vi "AlliGator Parameter Map Actions.vi"(0 "AlliGator Q Elements in":T6[](array[typedef]), 1 "VI in":refnum<vi>, 2 "Script in":bool, 5 "data value reference":refnum<data-value>, 7 "AlliGator Q Event in":T7=enum."GUI:Idle", 9 "Data":variant, 11 "error in (no error)":errorcluster, 12 "AlliGator Ctrl Refnums":T8) -> (3 "Script out":bool, 4 "AlliGator Q Elements out":T6[](array[typedef]), 6 "Data Value Reference out":refnum<data-value>, 10 "[Notebook Message]":T1[](array[typedef]) {"Message Style"."Font Size" min=6.0 step=1.0}, 15 "error out":errorcluster)   [LabVIEW 2021, in "AlliGator Action Engine.lvlib"]
doc: "Processes AlliGator decay fit parameter map-related actions."
uses:
  AlliGator Action Engine.lvlib
  Internal Variables/AlliGator Internal Variables v2.ctl
  <vilib>/vision/Image Controls.llb/IMAQ Image.ctl
  Internal Variables/AlliGator Gate Image Set.ctl
  Files/AlliGator FLI Dataset Type.ctl
  Files/AlliGator Data Series Type.ctl
  Dual-Channel Datasets/AlliGator Dataset Channel.ctl
  Settings/AlliGator Gate Arithmetic.ctl
  Source Image/AlliGator Displayed Image.ctl
  Image/Named ROI Description.ctl
  Phasor Graph/AlliGator Decay Metadata v3.ctl
  Decay Analysis/Decay Preprocessing/AlliGator Decay Background Subtraction Info.ctl
  Decay Analysis/Decay Preprocessing/AlliGator Baseline Subtraction Method.ctl
  Graphs/XY Graph/XY Graph Plot Shift Parameters.ctl
  Graphs/XY Graph/XY Graph Plot Shift Method.ctl
  Decay Analysis/Decay Preprocessing/AlliGator Decay Extrapolation Parameters.ctl
  Phasor/Calibration Phasor (m, phi).ctl
  Phasor/Phasor Reference Series.ctl
  Phasor/Phasor Calibration Map v2.ctl
  Phasor/Phasor (g, s).ctl
  Phasor Graph/AlliGator Raw Phasor Plot Data v5.ctl
  Phasor/Phasor Standard Deviation Options.ctl
  Phasor Plot/AlliGator Phasor Multi-Harmonic Data.ctl
  Phasor/Phasor Harmonic Data.ctl
  Decay Fit Parameter Map/AlliGator Decay Fit Options & Parameters v4.ctl
  Fits/IRF(X)PSED/Decay Fit Options v4.ctl
  Fits/Decay Convolution/Decay Model.ctl
  Fits/Residual Type.ctl
  Fits/IRF(X)PSED/Fit Weights Type v2.ctl
  Fits/Non-linear Fitting Method v2.ctl
  Fits/Fit Calculation Method.ctl
  Fits/Non-linear Fitting Algorithm.ctl
  Decay Analysis/Decay Fit/AlliGator Decay Fit Parameter Constraints 2.ctl
  Fits/IRF(X)PSED/Decay Fit Parameters In List.ctl
  Fits/IRF(X)PSED/MLE Baseline Offset Type.ctl
  Decay Analysis/Decay Preprocessing/AlliGator Decay Preprocessing Parameters.ctl
  Fits/IRF(X)PSED/Decay Fit Parameters & Derived Quantities List v2.ctl
  Fits/IRF(X)PSED/Decay Fit Result Constraint.ctl
  Decay Fit Parameter Map/AlliGator Parameter Maps Data.ctl
  AlliGator Q Event.ctl
  GUI/AlliGator Ctrl Refnums.ctl
  GUI/AlliGator Other Ctrl Refnums.ctl
  GUI/AlliGator State Indicator.ctl
  GUI/AlliGator Main Window Tabs.ctl
  GUI/AlliGator Phasor Plot Ctrl Refnums.ctl
  GUI/AlliGator Phasor Graph Ctrl Refnums.ctl
  Phasor/Phasor Calibration Type.ctl
  GUI/AlliGator Dataset Ctrl Refnums.ctl
  GUI/AlliGator Registered Events Ctrl Refnums.ctl
  GUI/AlliGator Image Histogram Control Refnums.ctl
  Histograms/Linear Histogram Options.ctl
  Histograms/Histogram Bin Option.ctl
  Histograms/Histogram Bin Position.ctl
  Decay Fit Parameter Map/AlliGator Decay Fit Map Control Refnums.ctl
  Parameter Map/AlliGator Parameter Map Control Refnums.ctl
  AlliGator Q Element.ctl
  Notebook/Notebook Message Object.ctl
  Rich Text Box/Text Formatting.ctl
  Rich Text Box/Text Colors.ctl
  Rich Text Box/Text Style.ctl
  Rich Text Box/Text Alignment.ctl
  Parameter Map/AlliGator New Parameter Map Set Event Data.ctl
  Alligator Elements Order in Action Stack.ctl
  Globals, Variables, Constants/AlliGator Variables List.ctl
  GUI/AlliGator Image Display Type.ctl
  Palette/Image Palette Information.ctl
  Image/Image Display Palette Type.ctl
  Utilities/Read-Write.ctl
  GUI/AlliGator Image Mouse Up Event Data.ctl
  Image/Image ROI Descriptor.ctl
  Image/Image Contour Definition.ctl
  Image/Image Contour ID.ctl
  Image/Image ROI Type.ctl
  Image/Image Control Refnum.ctl
  Rich Text Box/Text Format List.ctl
  c5217346-0728-4db9-a30e-52dae72b7cfc.vi
  AlliGator Add Single Action to Stack.vi
  Variant/Variant to Data/Variant to [String].vi
  Variant/Variant to Data/Variant to String.vi
  Variant/Variant to Data/Variant to Boolean.vi
  Variant/Variant to Data/Variant to I32.vi
  Variant/Variant to Data/Variant to U16.vi
  GUI/GUI.lvlib
  Variant/Variant to Data/Variant to Data.lvlib
  Globals, Variables, Constants/AlliGator Globals, Variables & Constants.lvlib
  Palette/Palette.lvlib
  GUI/AlliGator GUI.lvlib
  Image/Image.lvlib
  Files/AlliGator Files.lvlib
  Internal Variables/AlliGator Internal Variables.lvlib
  Files/Load-Save File Info.ctl
  Files/Files.lvlib
  Decay Fit Parameter Map/AlliGator Decay Fit Parameter Map.lvlib
  Sound/Sound.lvlib
  Parameter Map/AlliGator Parameter Map.lvlib
  Local Decay Window/AlliGator Local Decay Window.lvlib
  Notebook/Notebook.lvlib
  Utilities/Utilities.lvlib
  Phasor/Phasor.lvlib
  Decay Analysis/Decay Preprocessing/AlliGator Decay Preprocessing.lvlib
  Graphs/XY Graph/XY Graph Add-Ons.lvlib
  Phasor Graph/AlliGator Phasor Graph.lvlib
  Phasor Plot/AlliGator Phasor Plot.lvlib
  Source Image/AlliGator Source Image.lvlib
  Fits/Fits.lvlib
  Decay Analysis/Decay Fit/AlliGator Decay Fit.lvlib
  Settings/AlliGator Settings.lvlib
  Rich Text Box/Rich Text Box.lvlib
  Dual-Channel Datasets/AlliGator Dual-Channel Datasets.lvlib
  Histograms/Histogram Window.lvlib
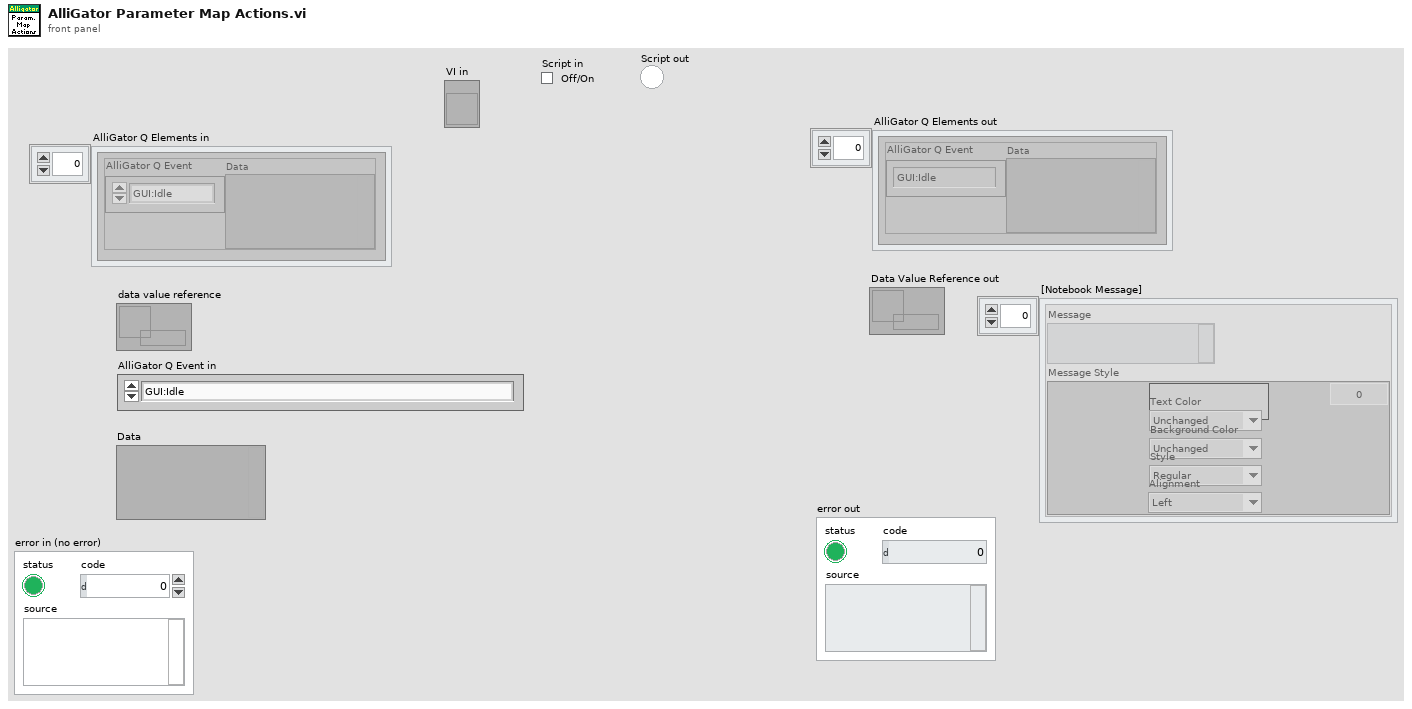
[diagram p1: front panel]
types:
  T1 = typedef "Notebook.lvlib/Notebook Message Object.ctl" = cluster{"Message":string, "Message Style":T2}
  T2 = typedef "Rich Text Box.lvlib/Text Formatting.ctl" = cluster{"Font":string, "Text Color":T3, "Background Color":T3, "Style":T4, "Font Size":dbl, "Alignment":T5}
  T3 = typedef "Rich Text Box.lvlib/Text Colors.ctl" = enum16{"Unchanged", "Black", "Blue", "Cyan", "Maroon", "Gray", "Violet", "Green", "Light Green", "Orange", "Yellow", "Magenta", "Red", "White"}
  T4 = typedef "Rich Text Box.lvlib/Text Style.ctl" = enum16{"Regular", "Bold", "Italic", "Underline", "Strikeout"}
  T5 = typedef "Rich Text Box.lvlib/Text Alignment.ctl" = enum16{"Left", "Right", "Center"}
  T6 = typedef "AlliGator Action Engine.lvlib/AlliGator Q Element.ctl" = cluster{"AlliGator Q Event":T7, "Data":variant}
  T7 = typedef "AlliGator Action Engine.lvlib/AlliGator Q Event.ctl" = enum16{"---- Files ----", "Files:Set Batch Export Files To Save", "Files:Set Dataset Loading & Pre-processing Options", "Files:Check #Frames in Dataset", "Files:Increment Frame Index", "Files:Open Mask Image", "Files:Open White Light Image", "Files:Open Single Dataset", "Files:New Folder of Folders Selected", "Files:Load File (all Types)_Scriptable", "Files:Move Flattened Series to Folders Series", "Files:Select Folder", "Files:Load FLI Dataset", "Files:Load Swiss SPAD 1 Dataset", "Files:Load Swiss SPAD 2 Dataset", "Files:Load .sdt FLI Dataset", "Files:Load .ptu FLI Dataset", "Files:Load .bin FLI Dataset", "Files:Load Single Gate Image Folder", "Files:Load I/m/phi Dataset (deprecated)", "Files:Load Single Image", "Files:Subtract Background File", "Files:Export FLI Dataset", "Files:Load HDF5 FLI Dataset", "Files:Set Destination File Path", "Files:Save Mask Image", "Files:Batch Conversion", "Files:New Folder Selected", "Files:Close FLI Dataset", "Files:Close FLI Dataset Series", "Files:Close White Light Image", "Files:Close Mask Image", "---- FLI Dataset ----", "FLI Dataset:Channel Arithmetic", "FLI Dataset:Export Average Lifetime Map as ASCII", "FLI Dataset:Export User-Defined Quantity Map as ASCII", "FLI Dataset:Python Function FLI Dataset Event", "FLI Dataset:ROI Analysis", "FLI Dataset:Tilted Logistic Square Gated IRF Characteristics Map", "FLI Dataset:Logistic Square Gated IRF Characteristics Map", "FLI Dataset:Square Gated IRF Characteristics Map", "FLI Dataset:Multi-ROI Single-Pixel Phasor Analysis", "FLI Dataset:Multi-ROI Single-Pixel NLSF Analysis", "FLI Dataset:All ROIs IRF Extraction", "FLI Dataset:All ROIs Decay Fit Non-Interactive (Fast + Individual IRF)", "FLI Dataset:All ROIs Phasor Analysis", "FLI Dataset:All ROIs Decay Fit", "FLI Dataset:Fluorescence Decay Statistics", "FLI Dataset:Update Decay Statistics Graph", "FLI Dataset:Get Decay from ROI", "FLI Dataset:All ROIs Average Lifetimes", "FLI Dataset:Save/Load Local IRFs", "FLI Dataset:Clear Local IRFs", "FLI Dataset:Phasor Calibration Maps (# Gates Series) Script", "FLI Dataset:Calibrated Phasor Map Series", "---- FLI Dataset Series ----", "FLI Dataset Series:Sum All Datasets in Series", "FLI Dataset Series:Add Dataset to Accumulated Dataset", "FLI Dataset Series:Display Accumulated Dataset", "FLI Dataset Series:Clear Dataset Series Sum", "FLI Dataset Series:Time-Series Analysis (NLSF)", "FLI Dataset Series:Time-Series Analysis (Phasor)", "---- Image ----", "Image:Update Image Profile Plots", "Image:Image Histogram Cursor Move", "Image:Image Histogram", "Image:Image Contrast", "Image:Set Image Histogram Cursor Move Flag", "Image:Clear Image Overlay", "Image:Use ROI as Search Area", "Image:Set ROI Diameter", "Image:Save Image Data as TIFF", "Image:Save Displayed Image with Overlay", "Image:Save Image Overlay Only", "Image:Save Image as Hot Pixel Mask", "Image:Change Source Image Color Palette", "Image:Copy Image to Clipboard", "Image:Source Image ROI Selection", "Image:Delete All ROIs", "Image:Delete All Unselected ROIs", "Image:Delete ROI", "Image:Merge All ROIs", "Image:Store ROI", "Image:Source Image ROI Storage", "Image:Export ROI Description to Notebook", "Image:Save ROI", "Image:Load ROI", "Image:Paste ROI Definition", "Image:Clear ROI", "Image:Identify ROIs in Mask Image", "Image:Create Complementary ROI", "Image:Create Contour ROI", "Image:Create ROI(s) from Pixels with Peak above Min_Scriptable", "Image:Create ROI(s) from Pixels with Intensity above Min_Scriptable", "Image:Compute ROI Statistics", "Image:Delete ROI(s) based on ROI Characteristics", "Image:Create ROI Grid", "Image:ROI to Individual Pixel ROIs", "Image:Python Function Source Image Event", "Image:Show Phasor Calibration Map ROI Centers", "Image:Convert ROI to Mask Image", "Image:Mouse Move", "Image:Mouse Up", "Image:Set Source Image Mouse Move Flag", "Image:Add Scale Bar Overlay", "Image:Delete Existing ROIs Option", "Image:Overlay ROI Median", "Image:Check Current ROI", "Image:Update True Pixel Value", "---- Decay ----", "Decay:Clear IRF/Reference Plot", "Decay:Add Decay to Graph", "Decay:Smoothen Plot", "Decay:Smoothen Plot Tail", "Decay:Average Selected Plots", "Decay:Extract IRF", "Decay:Optimal IRF Extraction", "Decay:Threshold IRF", "Decay:Fit to Model IRF", "Decay:Fit IRF to Square Gate", "Decay:Fit IRF to Logistic Square Gate", "Decay:Fit IRF to Tilted Logistic Square Gate", "Decay:Create Bounding Cursors Set", "Decay:Export Bounding Cursors Definition to Notebook", "Decay:Denoise Plot", "Decay:Compute Cumulative Function", "Decay:Use as Reference Decay", "Decay:Show Reference Decay/IRF", "Decay:Extrapolate Decay", "Decay:Create Head & Tail Bounding Cursors", "Decay:Store Cursor-defined Head & Tail Fractions", "Decay:Rebin Plot", "Decay:1-Normalize Decay", "Decay:[0-1]-Normalize Plot", "Decay:Straighten Decay", "Decay:Shift Decay", "Decay:Fold Decay", "Decay:Fit Decay", "Decay:Global Fit of Selected Decays", "Decay:Post Global Fit Script", "Decay:Add Global Fit Parameters to Graph", "Decay:Add Decay Parameter(s) to Plot (Graph)", "Decay:Export Decay to Phasor Graph", "Decay:Compute Average Lifetime", "Decay:Plot Convolution", "Decay:Graph Tip Strip Update", "---- Decay Statistics ----", "Decay Statistics:Tip Strip Update", "---- Intensity Time Trace ----", "Intensity Time Trace:Use File Timestamp", "Intensity Time Trace:Load Intensity Corrections File", "Intensity Time Trace:Clear Intensity Corrections File", "Intensity Time Trace:Tip Strip Update", "---- Phasor Plot ----", "Phasor Plot:Build Phasor Plot", "Phasor Plot:Change Phasor Plot Color Palette", "Phasor Plot:Adjust Phasor Plot Display Range", "Phasor Plot:Highlight Image ROI in Phasor Plot", "Phasor Plot:Save Phasor Plot Image with Overlay", "Phasor Plot:Export Complex Phasor Map", "Phasor Plot:Export Phasor Ratio Map", "Phasor Plot:Export Average Lifetime Map", "Phasor Plot:Compute Phase Lifetime Histogram", "Phasor Plot:Compute Phasor Ratio Histogram", "Phasor Plot:Compute Phase Lifetime vs Intensity Scatter Plot", "Phasor Plot:Weber 2-Component Decomposition", "Phasor Plot:Update Phasor Color Map Vertices", "Phasor Plot:Clear Phasor Overlay", "Phasor Plot:Use Segment Extremities as References", "Phasor Plot:Use UC/Segment Intersections as References", "Phasor Plot:Use UC/Principal Axis Intersections as References", "Phasor Plot:Use UC/Linear Fit Intersections as References", "Phasor Plot:Update Phasor Plot Reference", "Phasor Plot:Show Local Phasor Info in Phasor Plot", "Phasor Plot:Update Phasor Plot State", "Phasor Plot:Phasor Plot ROI Storage", "Phasor Plot:Phasor Plot ROI Selection", "Phasor Plot:Python Function Phasor Plot Event", "Phasor Plot:Overlay Phasor ROI, Ratio or Map in Source Image", "Phasor Plot:Compute Decay of Selected Phasors", "Phasor Plot:Phasor at Image Pixel", "Phasor Plot:Mouse Move", "Phasor Plot:Mouse Up", "Phasor Plot:Display Range Mouse Move", "Phasor Plot:Set Mouse Move Flag", "Phasor Plot:Update True Phasor Plot Value", "---- Phasor Graph ----", "Phasor Graph:Get Phasor Value", "Phasor Graph:Create New Phasor Plot Dialog", "Phasor Graph:Update Last Phasor Value", "Phasor Graph:Update Phasor (m, phi)", "Phasor Graph:Remove Single Phasor from Plot", "Phasor Graph:Add Single Phasor to Plot", "Phasor Graph:Remove Phasor Plot", "Phasor Graph:Remove Selected Phasor Plots", "Phasor Graph:Clear Phasor Data", "Phasor Graph:Clear Phasor Graph", "Phasor Graph:Cursor Move", "Phasor Graph:Draw Cursor Connecting Line", "Phasor Graph:Clear Cursor Connecting Line", "Phasor Graph:Find UC Intersection", "Phasor Graph:Use UC/Cursor-Defined Line Intersections", "Phasor Graph:Use Selected Plots Fitted Line/UC Intersections", "Phasor Graph:Use Selected Plots Principal Axis/UC Intersections", "Phasor Graph:Show Single Phasor", "Phasor Graph:Save Single Phasor Plot", "Phasor Graph:Save All Phasor Plots", "Phasor Graph:Load Phasor Plot(s)", "Phasor Graph:Phasor Multiplication", "Phasor Graph:Compute Average Phasor", "Phasor Graph:Compute Multiple Average Phasors (Selected Plots)", "Phasor Graph:Export Single Phasor Plot Phase Lifetimes", "Phasor Graph:Parameter 2 vs Parameter 1 Scatter Plot", "Phasor Graph:Use Cursor n Location", "Phasor Graph:Set Reference n to Current Phase Lifetime Value", "Phasor Graph:Set Reference n to Lifetime Value", "Phasor Graph:Set Cursor n Location", "Phasor Graph:Save Phasor Graph Image", "Phasor Graph:Update SEPL Plot", "Phasor Graph:Export Single Phasor Plot Data", "Phasor Graph:Export Selected Phasor Plots Data", "Phasor Graph:Python Function Phasor Graph Event", "Phasor Graph:Tip Strip Update", "---- Calibration ----", "Calibration:Set Calibration Type", "Calibration:Load/Save Phasor Calibration", "Calibration:Load/Save Phasor Calibration Series", "Calibration:Load/Save Phasor Calibration Map", "Calibration:Use as Calibration", "Calibration:Compute Optimal Calibration from Phasor References", "Calibration:Clear Phasor Calibration", "Calibration:Single Phasor Calibration Information", "Calibration:Use as Calibration Series", "Calibration:Use as Calibration Map", "Calibration:Clear Calibration Series", "Calibration:Phasor Calibration Series Information", "Calibration:Clear Calibration Map", "Calibration:Phasor Calibration Map Information", "Calibration:Apply Phasor Calibration", "Calibration:Update Single Plot Calibration", "Calibration:Update Multiple Plots Calibration", "Calibration:Clear Single Plot Calibration", "Calibration:Clear All Plots Calibrations", "Calibration:Clear Plot(s) Calibration(s)?", "---- Phasor Ratio ----", "Phasor Ratio:Clear Reference n", "Phasor Ratio:Toggle Selected Plot(s)  Lock to Reference 1", "Phasor Ratio:Use as Reference n", "Phasor Ratio:Send Reference n to Notebook", "Phasor Ratio:Toggle Selected Plot(s)  Lock to Reference 2", "Phasor Ratio:Compute Phasor Ratio at Mouse Location", "Phasor Ratio:Compute Phasor Plot's Average Phasor Ratio", "Phasor Ratio:Compute Time-Series Phasor Ratios", "Phasor Ratio:Fit Line to Phasor Ratio Plot", "Phasor Ratio:Save References", "Phasor Ratio:Load References", "Phasor Ratio:Update Phasor Reference 1", "Phasor Ratio:Update Phasor Reference 2", "Phasor Ratio:Move Cursor n to Reference n", "Phasor Ratio:Use as Phasor Reference 1 Lifetime", "Phasor Ratio:Use as Phasor Reference 2 Lifetime", "Phasor Ratio:Export Phasor Ratio Map as ASCII", "Phasor Ratio:Tip Strip Update", "---- Lifetime & Other Parameters Graph ----", "Lifetime:Compute Sliced Mean, SDV and CV Plots", "Lifetime:Plot Decay Shifts", "Lifetime:Plot Histogram", "---- Decay Fit Parameter Map ----", "Decay Fit Parameter Map:Export ROI NLSF Data as ASCII", "Decay Fit Parameter Map:Set Decay Fit Parameter Map Selection", "Decay Fit Parameter Map:Build Decay Fit Parameter Map", "Decay Fit Parameter Map:Change Decay Fit Parameter Map Color Palette", "Decay Fit Parameter Map:Export Decay Fit Parameter Map Data as ASCII", "Decay Fit Parameter Map:Export All Decay Fit Parameter Maps Data as ASCII", "Decay Fit Parameter Map:Selected Parameter Scatterplot", "Decay Fit Parameter Map:Parameter 2 vs Parameter 1 Scatterplot", "Decay Fit Parameter Map:Save Decay Fit Parameter Map Image", "Decay Fit Parameter Map:Save-Load IRFs & Fit Data", "Decay Fit Parameter Map:Update Local Decay Plots", "Decay Fit Parameter Map:Python Function Decay Fit Parameters Map Event", "Decay Fit Parameter Map:Overlay Decay Fit Parameter Map in Source Image", "Decay Fit Parameter Map:Selected Parameter vs Intensity Scatterplot", "Decay Fit Parameter Map:Mouse Up", "Decay Fit Parameter Map:Mouse Move", "Decay Fit Parameter Map:Display Range Mouse Move", "Decay Fit Parameter Map:Change Map Resolution", "Decay Fit Parameter Map:Variance Significance Maps", "Decay Fit Parameter Map:Fit Result Constraints Window", "---- Parameter Map ----", "Parameter Map:Export ROI Parameters Data as ASCII", "Parameter Map:Add Parameter Map Set", "Parameter Map:Delete Parameter Map Set", "Parameter Map:Update Parameter List", "Parameter Map:Build Parameter Map", "Parameter Map:Change Parameter Map Color Palette", "Parameter Map:Export Parameter Map Data as ASCII", "Parameter Map:Export All Parameter Maps Data as ASCII", "Parameter Map:Selected Parameter Scatterplot", "Parameter Map:Parameter 2 vs Parameter 1 Scatterplot", "Parameter Map:Selected Parameter vs Intensity Scatterplot", "Parameter Map:Save Parameter Map Image", "Parameter Map:Save-Load IRFs & Parameter Maps (TODO)", "Parameter Map:Set Parameter Map Selection", "Parameter Map:Python Function Parameter Map Event", "Parameter Map:Overlay Parameter Map in Source Image", "Parameter Map:Update Local Decay Plots", "Parameter Map:Mouse Up", "Parameter Map:Mouse Move", "Parameter Map:Display Range Mouse Move", "---- Generic Graph ----", "Generic Graph:Generic XY Graph Event", "Generic Graph:Python Function XY Graph Event", "Generic Graph:New Plot", "Generic Graph:Save Plot", "Generic Graph:XY Plot Histogram", "Generic Graph:Set XY Graph Plot Name", "Generic Graph:Set Last Cursor Style", "Generic Graph:Tip Strip Update", "---- GUI ----", "GUI:Start Script", "GUI:Type of Displayed Image Changed", "GUI:Gate Image Slide Changed", "GUI:Show Busy Icon", "GUI:Show Busy Icon & Abort Button", "GUI:Hide Busy Icon", "GUI:Hide Busy Icon & Abort Button", "GUI:Abort", "GUI:End Script", "GUI:Start Timing", "GUI:End Timing", "GUI:Set State Indicator", "GUI:Send Parameters JSON Strings to Clipboard", "GUI:Set Gate Step", "GUI:Idle", "GUI:Initialization", "GUI:Quit", "GUI:Increment Dataset Index", "GUI:Set Dataset Index to -1", "GUI:Time Series Slider Moved", "GUI:Time Series Slider Changed", "GUI:Toggle Playback or Loop", "GUI:Playback Script", "GUI:Set Phasor Frequency", "GUI:Open Window", "GUI:Start Test Script", "GUI:End Test Script", "GUI:Set Verbose Mode", "GUI:Set Verbose Settings Mode", "DEBUG"}
  T8 = typedef "AlliGator GUI.lvlib/AlliGator Ctrl Refnums.ctl" = cluster{"Other AlliGator Ctrl Refnums":T9, "Phasor Plot Ctrl Refnums":T10, "Phasor Graph Ctrl Refnums":T11, "Dataset Control Refnums":T12, "Registered Events Ctrl Refnums":T13, "Image Histogram Ctrl Refnums":T14, "Decay Fit Map Ctrl Refnums":T15, "Parameter Map Ctrl Refnums":T16}
  T9 = typedef "AlliGator GUI.lvlib/AlliGator Other Ctrl Refnums.ctl" = cluster{"State Indicators":refnum<vi>, " Progress Bar":refnum<vi>, "Decay Graph Active":refnum<vi>, "Decay Statistics Bin":refnum<vi>, "Time Step":refnum<vi>, "Use File Timestamp":refnum<vi>, "Tab Control":refnum<vi>, "CPU":refnum<vi>, "Abort Fit":refnum<vi>, "Dataset File/Folder Path":refnum<vi>, "Abort ROI Creation":refnum<vi>, "Event LED":refnum<vi>, "Dataset File/Folder Path 2":refnum<vi>, "Dataset File/Folder Path 3":refnum<vi>, "Dataset File/Folder Path 4":refnum<vi>, "Dataset File/Folder Path 5":refnum<vi>, "Dataset File/Folder Path 6":refnum<vi>, "Dataset File/Folder Path 7":refnum<vi>, "Dataset File/Folder Path 8":refnum<vi>, "Dataset File/Folder Path 9":refnum<vi>, "Dataset File/Folder Path 10":refnum<vi>, "Dataset File/Folder Path 11":refnum<vi>}
  T10 = typedef "AlliGator GUI.lvlib/AlliGator Phasor Plot Ctrl Refnums.ctl" = cluster{"Phasor Ratio":refnum<vi>, "Modulus Lifetime":refnum<vi>, "Phasor at cursor (m, phi)":refnum<vi>, "Phase Lifetime":refnum<vi>, "Phasor at cursor (g, s)":refnum<vi>, "Phasor Plor Average Lifetime":refnum<vi>, "Phasor Plot Active":refnum<vi>, "Save Phasor Plot":refnum<vi>, "Image Overlay Color":refnum<vi>, "Phasor Plot Color Scale":refnum<vi>, "Reference 1 Button":refnum<vi>, "Reference 2 Button":refnum<vi>, "True Phasor Plot Value":refnum<vi>}
  T11 = typedef "AlliGator GUI.lvlib/AlliGator Phasor Graph Ctrl Refnums.ctl" = cluster{"Phasor Ratio":refnum<vi>, "Modulus Lifetime":refnum<vi>, "Phasor at cursor (m, phi)":refnum<vi>, "Phase Lifetime":refnum<vi>, "Phasor at cursor (g, s)":refnum<vi>, "Phasor Graph Average Lifetime":refnum<vi>, "Phasor Graph Active":refnum<vi>, "Save Phasor Graph":refnum<vi>, "Phasor Frame Slide":refnum<vi>, "Single Step Phasor":refnum<vi>, "Calibration Type":refnum<vi>, "Show Line":refnum<vi>, "Phase Lifetime 1":refnum<vi>, "Phase Lifetime 2":refnum<vi>, "Phasor Graph Frequency":refnum<vi>, "Phasor Reference 1 Control":refnum<vi>, "Phasor Reference 2 Control":refnum<vi>, "Calibration Lifetime":refnum<vi>, "Phase Lifetime SDV":refnum<vi>, "Average Lifetime SDV":refnum<vi>, "Phasor Ratio SDV":refnum<vi>, "Modulus Lifetime SDV":refnum<vi>}
  T12 = typedef "AlliGator GUI.lvlib/AlliGator Dataset Ctrl Refnums.ctl" = cluster{"Current Data":refnum<vi>, "Gate Image Slide":refnum<vi>, "Time Point Slide":refnum<vi>, "Current Time Stamp":refnum<vi>, "Save Image":refnum<vi>, "Displayed Image":refnum<vi>, "Overlay Mode":refnum<vi>, "Phasor Overlay Color":refnum<vi>, "Image Color Scale":refnum<vi>, "Use ROI as Search Area":refnum<vi>, "Source Image ROI Color":refnum<vi>, "True Pixel Value":refnum<vi>}
  T13 = typedef "AlliGator GUI.lvlib/AlliGator Registered Events Ctrl Refnums.ctl" = cluster{"Time Point Slider":refnum<vi>, "Phasor Plot Display Range":refnum<vi>, "Decay Graph":refnum<vi>, "Decay Statistics Graph":refnum<vi>, "Intensity Time Trace":refnum<vi>, "Phasor Graph":refnum<vi>, "Phasor Ratio Graph":refnum<vi>, "Lifetime Graph":refnum<vi>, "Phasor Plot Display":refnum<vi>, "Source Image Display":refnum<vi>, "Decay Fit Parameter Map Display Range":refnum<vi>, "Decay Fit Parameter Map Display":refnum<vi>, "Parameter Map Display Range":refnum<vi>, "Parameter Map Display":refnum<vi>, "Phasor Plot Display Range":refnum<vi>}
  T14 = typedef "AlliGator GUI.lvlib/AlliGator Image Histogram Control Refnums.ctl" = cluster{"Image Histogram":refnum<vi>, "Image Histogram Options":refnum<vi>, "Image Histogram Active":refnum<vi>, "Image Histogram Upper Percentile":refnum<vi>, "Image Histogram Lower Percentile":refnum<vi>, "Auto-Adjust Contrast":refnum<vi>}
  T15 = typedef "AlliGator Decay Fit Parameter Map.lvlib/AlliGator Decay Fit Map Control Refnums.ctl" = cluster{"Decay Fit Parameter Map Color Scale":refnum<vi>, "Decay Fit Parameter":refnum<vi>, "Max Parameter":refnum<vi>, "Min Parameter":refnum<vi>, "Decay Fit Parameter Map Display":refnum<vi>, "Decay Fit Parameter Map Display Range":refnum<vi>, "Decay Parameter Map X":refnum<vi>, "Decay Parameter Map Y":refnum<vi>, "Decay Parameter Map Value":refnum<vi>}
  T16 = typedef "AlliGator Parameter Map.lvlib/AlliGator Parameter Map Control Refnums.ctl" = cluster{"Parameter Map Color Scale":refnum<vi>, "Map Parameter":refnum<vi>, "Max Parameter":refnum<vi>, "Min Parameter":refnum<vi>, "Parameter Map Display":refnum<vi>, "Parameter Map Display Range":refnum<vi>, "Parameter Map Set":refnum<vi>, "Parameter Map X":refnum<vi>, "Parameter Map Y":refnum<vi>, "Parameter Map Value":refnum<vi>}
  T17 = typedef "AlliGator Action Engine.lvlib/Alligator Elements Order in Action Stack.ctl" = enum16{"Enqueue 2 AFTER 1", "Enqueue 2 BEFORE 1"}
  T18 = typedef "AlliGator Parameter Map.lvlib/AlliGator New Parameter Map Set Event Data.ctl" = cluster{"New Parameter Set Name":string, "Parameter Map Names":string[]}
  T19 = typedef "AlliGator GUI.lvlib/AlliGator Image Display Type.ctl" = enum16{"Source Image", "Phasor Plot", "Decay Fit Parameter Map", "Parameter Map"}
  T20 = typedef "AlliGator Globals, Variables & Constants.lvlib/AlliGator Variables List.ctl" = enum16{"---- GUI ----", "GUI:Initialization Status", "GUI:State Indicators Refnum", "GUI:Original AlliGator Menu Items", "GUI:Current Action Loop State", "GUI:Script in progress", "GUI:Playback", "GUI:Loop Playback", "GUI:Search ROI Used", "GUI:Search ROI", "Decay Graph Max Legend Size", "Intensity Graph Max Legend Size", "Decay Statistics Graph Max Legend Size", "Phasor Graph Max Legend Size", "Phasor Ratio Graph Max Legend Size", "Lifetime Graph Max Legend Size", "---- Files ----", "Files:Export Dataset Frames as Individual Files", "Files:Show Batch Export Help Balloons", "Files:Frames in Dataset", "Files:ptu File Frame Start Indices", "Files:Current Frame in Dataset", "Files:Current Frame Timestamp", "Files:Dataset Loaded", "Files:Dataset Metadata", "Files:Dataset Channel", "Files:Dataset Data Description", "Files:Background Dataset Metadata", "Files:Background Dataset Channel", "Files:Background Dataset Data Description", "Files:Background File Subtraction", "Files:Background File Path", "Files:Background File Pile-up Correction", "Files:Background File Pixel Well Capacity", "Files:Background File Scaling Factor", "Files:Current Dataset Load Settings", "Files:Dataset Path", "Files:ICCD-specific Information", "Files:Macrotime Gate Separation", "------ Python Plugins ------", "Python Plugins:Information", "Python Plugins:Python Session", "Python Plugins:Valid Python Session?", "---- Source Image ----", "Source Image:ROIs", "Source Image:Current ROI", "Source Image:ROI Event Refnum", "X_Source Image:Display Range", "X_Source Image:Palette Information", "X_Source Image:Type of Displayed Image", "X_Time Gate Slider", "Source Image:Palette List", "Source Image:Scale", "Source Image:ROI Overlay Color", "Source Image:Overlay to Erase", "Source Image:Is Displayed Image Accumulated", "Source Image:White Light Image Modified", "Source Image:Mask Image Modified", "---- Image Profile Window ----", "Image Profile:Window Event Refnum", "Image Profile:IntensityType", "Image Profile:Intensity Average Type", "Image Profile:Intensity-weighted SDV", "Image Profile:Box Profile Type", "Image Profile:Window Open", "Image Profile:Plotted Fit Parameter", "------ Phasor Graph -------", "Phasor Graph:Show Line", "---- Phasor Plot ---", "Phasor Plot:Parameters Changed", "Phasor Plot:FLI Dataset Modified since last Calculation", "Phasor Harmonics Data", "Selected Phasor Harmonics", "Phasor Harmonic Manager Event Refnum", "Phasor Plot:ROIs", "Phasor Plot:Current ROI", "Phasor Plot:ROI Event Refnum", "Phasor Plot:Image Reference Points", "Phasor Plot:Computed", "Phasor Plot:Palette Information", "Phasor Plot:Palette List", "Phasor Plot:Phasor Ratio Palette Information", "Phasor Plot:Phasor Ratio Palette List", "Phasor Plot:Image Scale", "Phasor Plot:Image Overlay to Erase", "Phasor Plot:Image Elements to Update", "Phasor Plot:Current Calculation Parameters", "Phasor Plot:Current Calibration Options", "Phasor Plot:Reset Cumulated Phasor Plot", "Phasor Plot:Reference 1", "Phasor Plot:Lifetime Reference 1", "Phasor Plot:Reference 1 Frequency", "Phasor Plot:Reference 2", "Phasor Plot:Lifetime Reference 2", "Phasor Plot:Reference 2 Frequency", "---- Decay Analysis ----", "Number of Selected Decays to Fit", "LS Fit Results", "LAR Fit Results", "BS Fit Results", "Last Decay Max - Min", "Best Fit Parameters", "Best Fit Parameter Names", "Actual Size X", "Actual Size Y", "Binning X", "Binning Y", "Actual # Gates", "Dataset Number", "Gates to...", "Gates Skipped", "Gates to keep", "Gate Step", "Gate Separation", "Reversed Gates", "Pile-up Correction", "Pixel Well Capacity", "Background Subtracted", "Background Subtraction Method", "Background Definition Range", "Background File (deprecated)", "Number of Dataset Accumulated", "Array of Accumulated Dataset Paths", "Do Averaged Datasets", "Destination File Path", "Process Plot Target", "Use 1/D as Phasor Frequency", "---- Decay Fit Parameter Map -----", "Decay Fit Parameter Map:Palette Information", "Decay Fit Parameter Map:Palette List", "Decay Fit Parameter Map:X Resolution", "Decay Fit Parameter Map:Y Resolution", "Decay Fit Parameter Map:Use Decay Fit Result Constraints", "Decay Fit Parameter Map:Decay Fit Result Constraints", "Decay Fit Parameter Map:Decay Fit Result Constraints Applied", "---- Parameter Map ----", "Parameter Map:Palette Information", "Parameter Map:Palette List", "------- Local Decay Window ---------", "Local Decay Graph Window:Event Refnum", "Local Decay Graph Window:Use normalized IRF for convolution", "----- Miscellaneous ----", "Misc:Skippable Dialog Windows Status"}
  T21 = typedef "Palette.lvlib/Image Palette Information.ctl" = cluster{"Palette Name [# Colors,int?,inv?]":string, "Palette Type":T22, "Palette Colors":u32[], "Interpolate?":bool}
  T22 = typedef "Image.lvlib/Image Display Palette Type.ctl" = u32
  T23 = typedef "Utilities.lvlib/Read-Write.ctl" = enum16{"Read", "Write"}
  T24 = typedef "AlliGator GUI.lvlib/AlliGator Image Mouse Up Event Data.ctl" = cluster{"Current ROI Tool":u32, "ROI Descriptor":T25, "Shift":bool, "Alt":bool, "Image Display Refnum":T29}
  T25 = typedef "Image.lvlib/Image ROI Descriptor.ctl" = cluster{"Global Rectangle":i32[], "Contours":T26[]}
  T26 = typedef "Image.lvlib/Image Contour Definition.ctl" = cluster{"Contour Type":T27, "ROI Type":T28, "Points":i32[]}
  T27 = typedef "Image.lvlib/Image Contour ID.ctl" = enum32{"External", "Internal"}
  T28 = typedef "Image.lvlib/Image ROI Type.ctl" = enum16{"No Selection", "Point", "Line", "Rectangle", "Oval", "Polygon", "Freehand Region", "Annulus", "Unused2", "Unused3", "Broken Line", "Freehand Line", "Rotated Rectangle"}
  T29 = typedef "Image.lvlib/Image Control Refnum.ctl" = refnum<vi>
  T30 = typedef "Notebook.lvlib/Text Format List.ctl" = enum16{"Message", "Result", "Error", "Setting", "Verbose", "Warning"}
  T31 = cluster{"Parameter Map Set":u16, "Map Parameter 1":u16, "Map Parameter 2":u16}
  T32 = typedef "Files.lvlib/Load-Save File Info.ctl" = cluster{"Load/Save":bool, "File Path":path}
  T33 = typedef "AlliGator Parameter Map.lvlib/AlliGator Parameter Map Update Event Data.ctl" = cluster{"Parameter":u16, "Parameter changed":bool, "Map Set":u16}
  T34 = typedef "AlliGator Parameter Map.lvlib/AlliGator Parameter Map Display Range Mouse Move Data.ctl" = cluster{"Parameter Map Set":u16, "Map Parameter":u16}
  T35 = typedef "Image.lvlib/Image Save File Format.ctl" = enum16{"PNG", "JPEG", "BMP"}
  T36 = typedef "ROI Descriptor" = cluster{"Global Rectangle":i32[], "Contours":cluster{"ID":enum32{"External", "Internal"}, "Type":u32, "Coordinates":i32[]}[]}
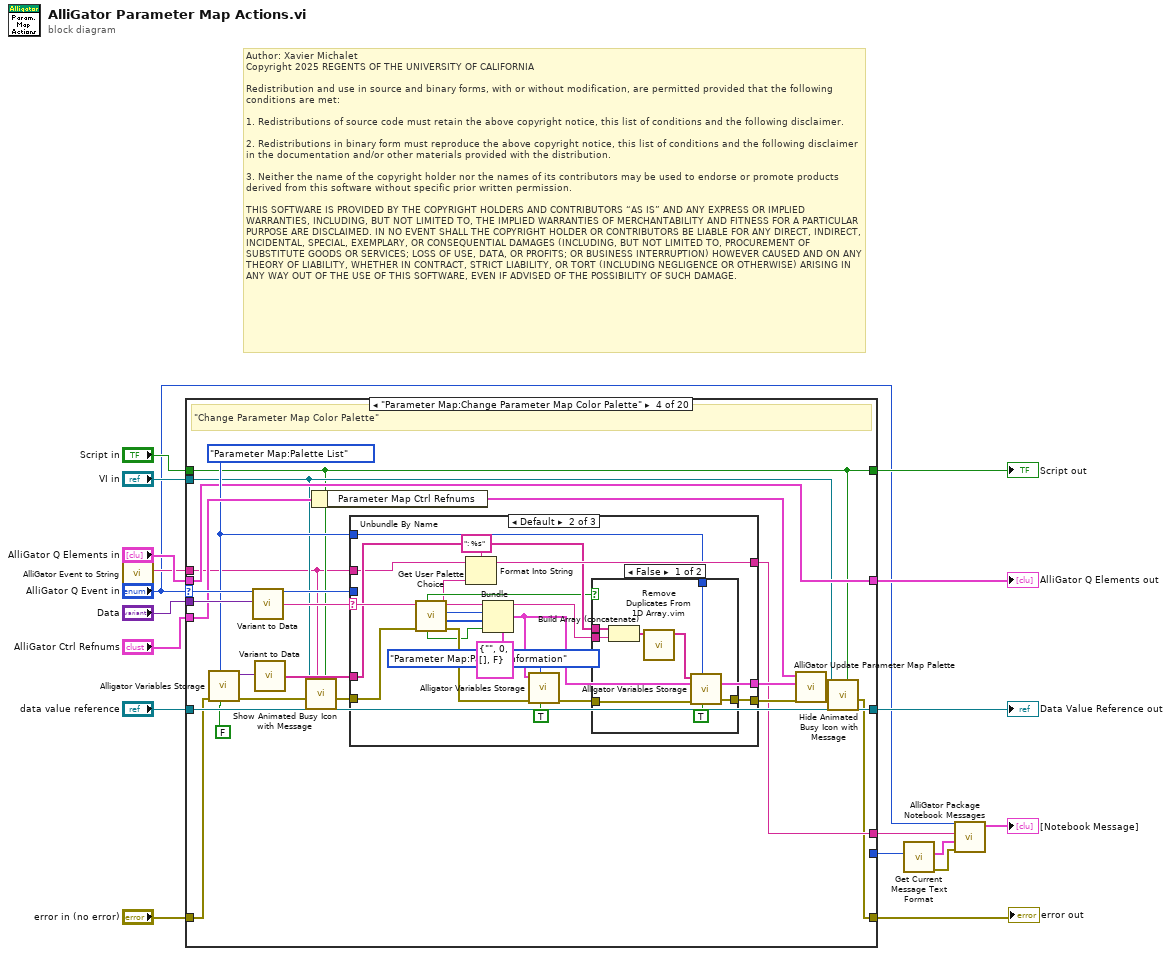
[diagram p0: block diagram]
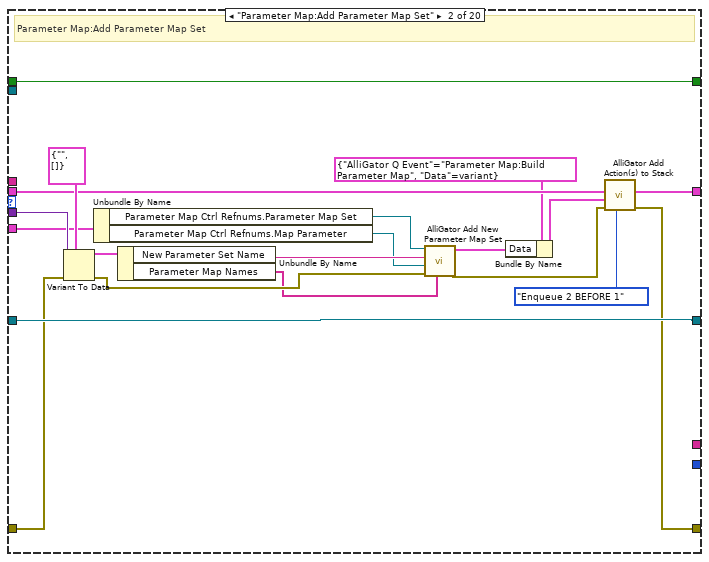
[diagram p3: hidden frame]
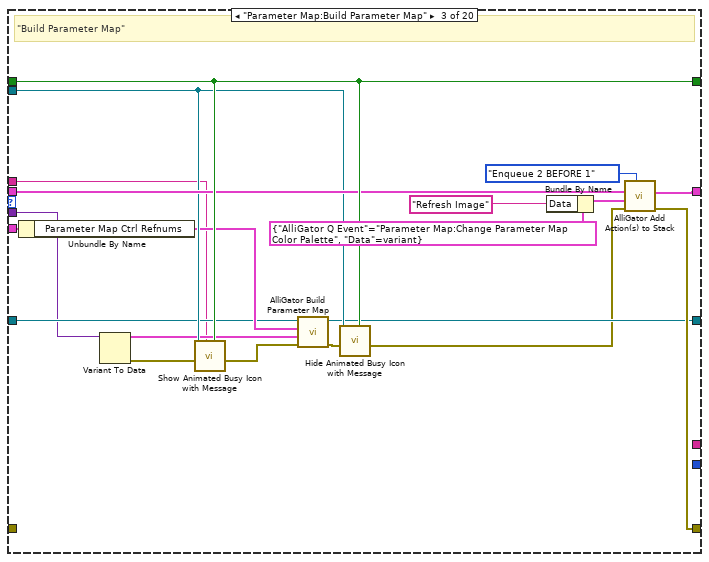
[diagram p4: hidden frame]
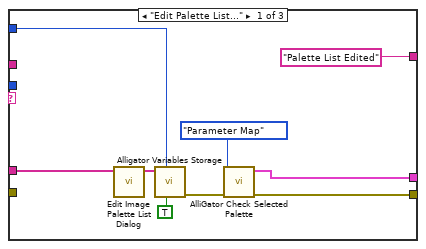
[diagram p5: hidden frame]
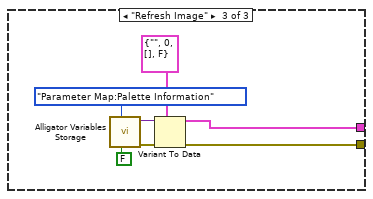
[diagram p7: hidden frame]
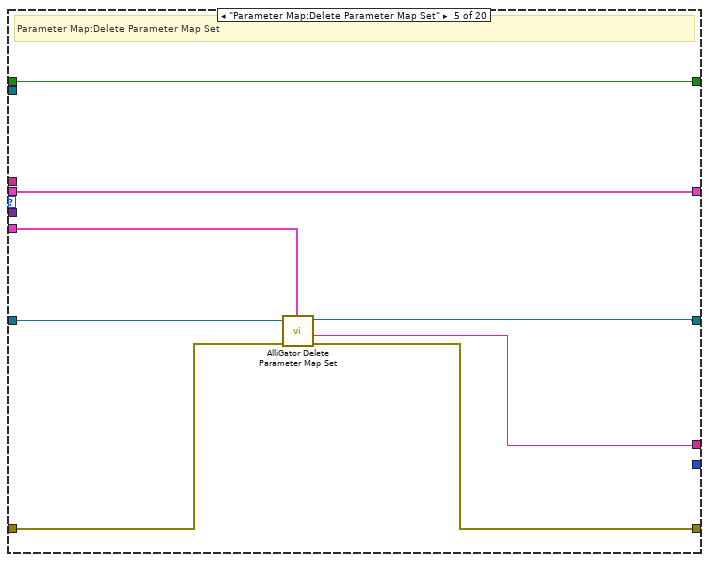
[diagram p8: hidden frame]
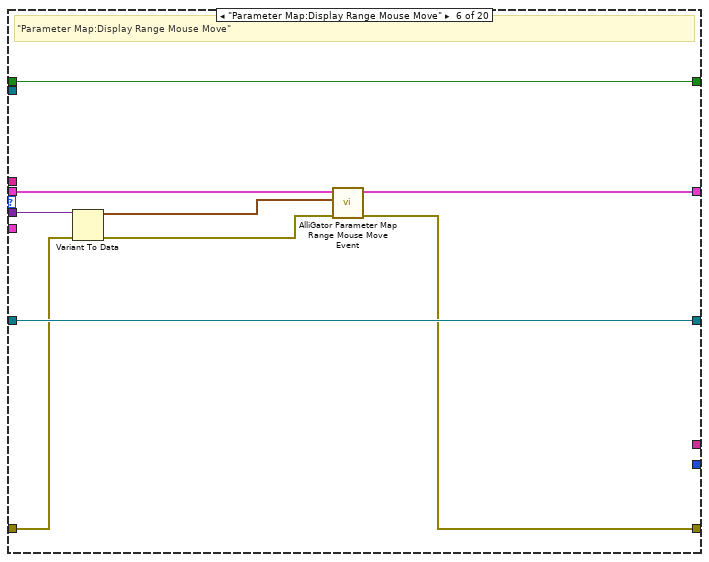
[diagram p9: hidden frame]
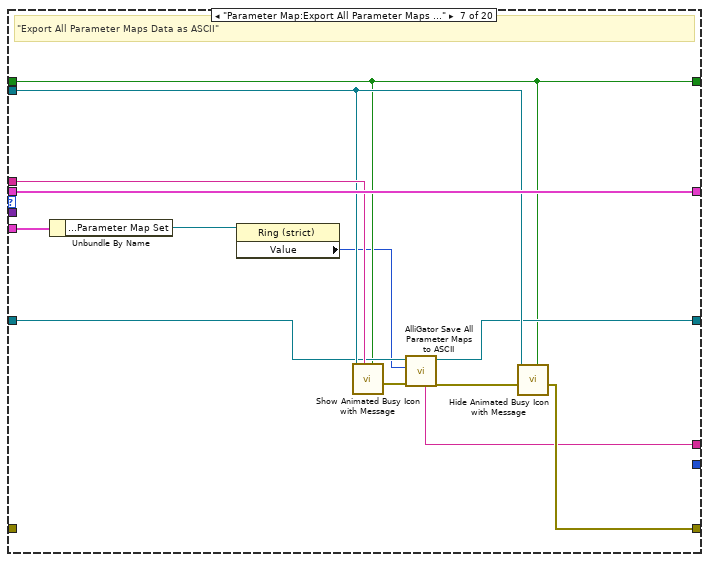
[diagram p10: hidden frame]
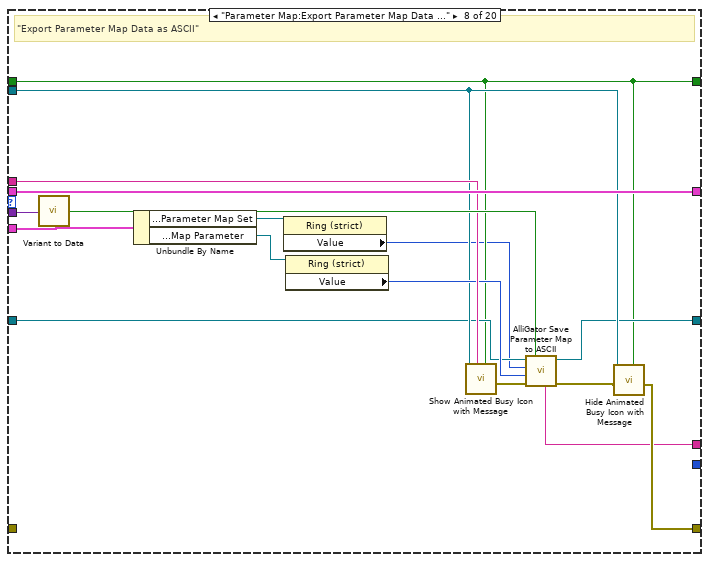
[diagram p11: hidden frame]
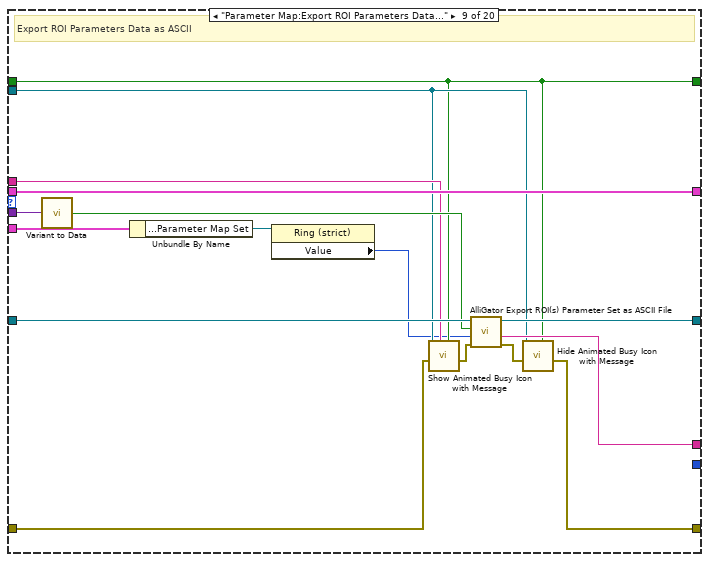
[diagram p12: hidden frame]
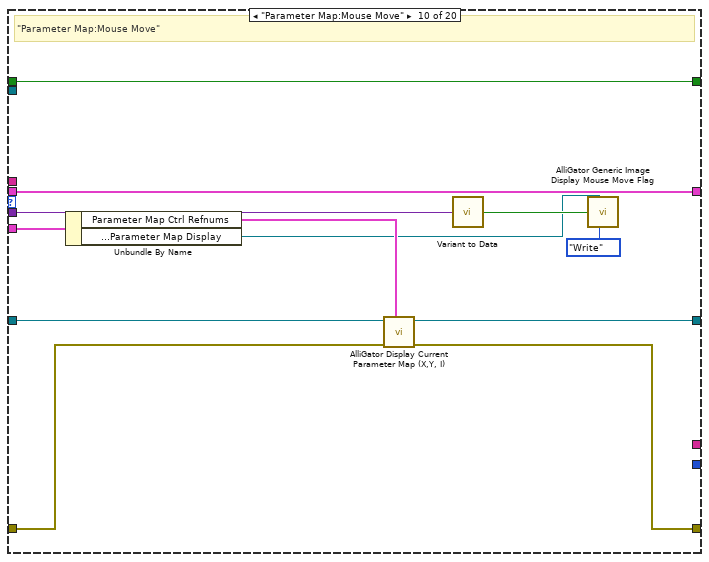
[diagram p13: hidden frame]
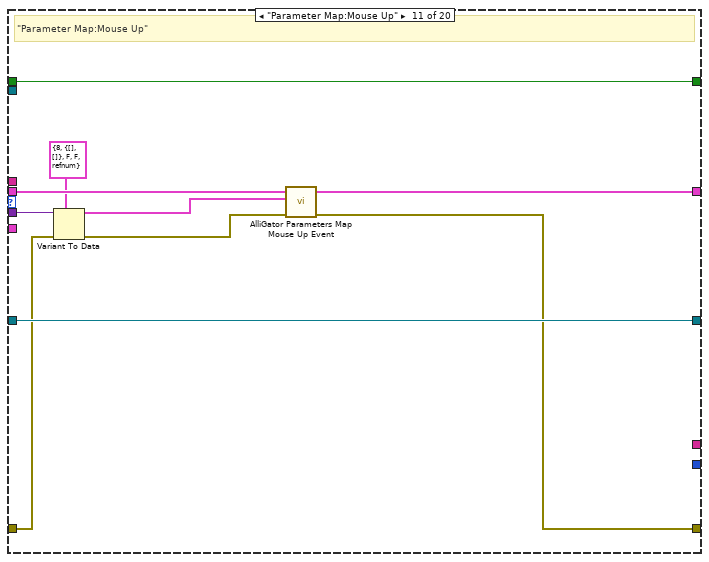
[diagram p14: hidden frame]
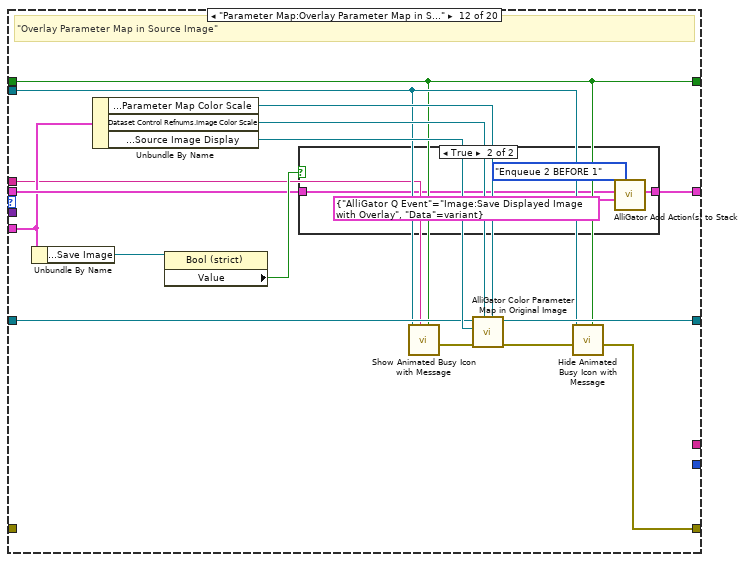
[diagram p15: hidden frame]
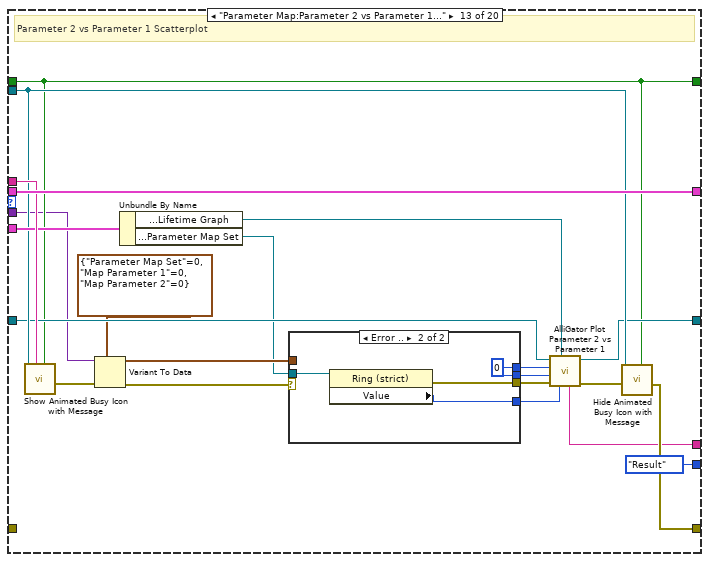
[diagram p17: hidden frame]
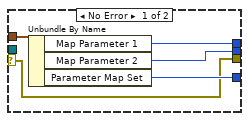
[diagram p18: hidden frame]
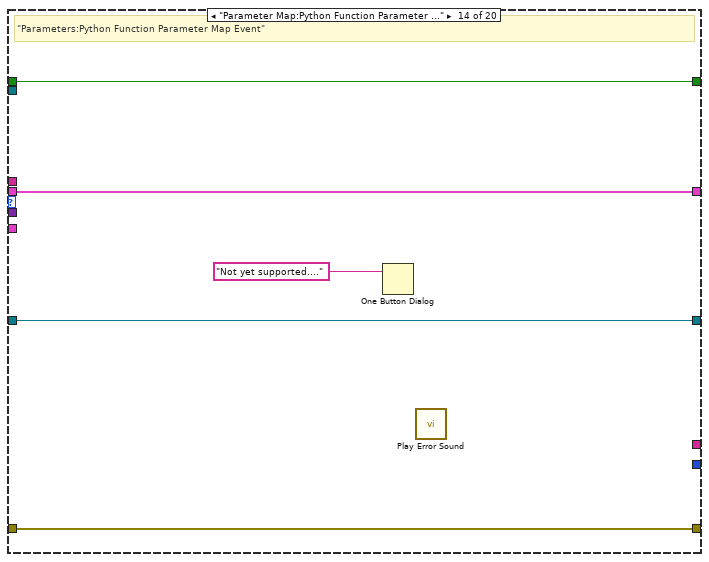
[diagram p19: hidden frame]
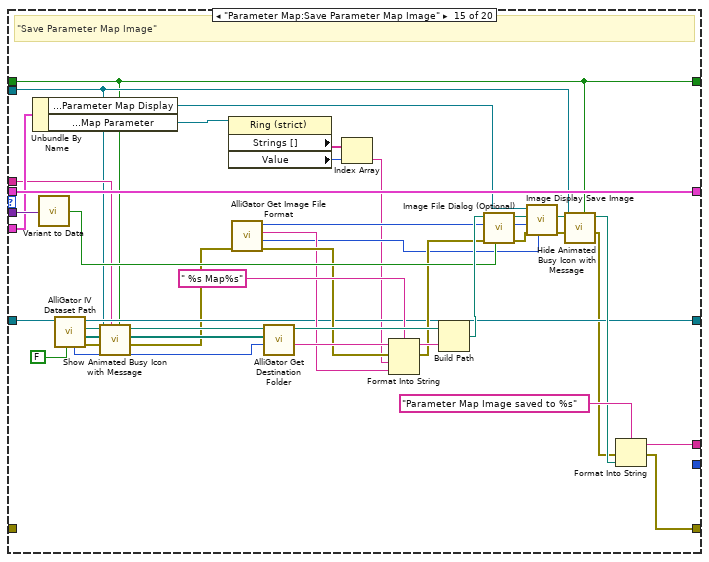
[diagram p20: hidden frame]
diagram:
  # "Author: Xavier Michalet\nCopyright 2025 REGENTS OF THE UNIVERSITY OF CALIFORNIA\n\nRedistribution and use in source and binary forms, with or without modification, are permitted provided that the following conditions are met:\n\n1. Redistributions of source code must retain the above copyright notice, this list of conditions and the following disclaimer.\n\n2. Redistributions in binary form must reproduce the above copyright notice, this list of conditions and the following disclaimer in the documentation and/or other materials provided with the distribution.\n\n3. Neither the name of the copyright holder nor the names of its contributors may be used to endorse or promote products derived from this software without specific prior written permission.\n\nTHIS SOFTWARE IS PROVIDED BY THE COPYRIGHT HOLDERS AND CONTRIBUTORS “AS IS” AND ANY EXPRESS OR IMPLIED WARRANTIES, INCLUDING, BUT NOT LIMITED TO, THE IMPLIED WARRANTIES OF MERCHANTABILITY AND FITNESS FOR A PARTICULAR PURPOSE ARE DISCLAIMED. IN NO EVENT SHALL THE COPYRIGHT HOLDER OR CONTRIBUTORS BE LIABLE FOR ANY DIRECT, INDIRECT, INCIDENTAL, SPECIAL, EXEMPLARY, OR CONSEQUENTIAL DAMAGES (INCLUDING, BUT NOT LIMITED TO, PROCUREMENT OF SUBSTITUTE GOODS OR SERVICES; LOSS OF USE, DATA, OR PROFITS; OR BUSINESS INTERRUPTION) HOWEVER CAUSED AND ON ANY THEORY OF LIABILITY, WHETHER IN CONTRACT, STRICT LIABILITY, OR TORT (INCLUDING NEGLIGENCE OR OTHERWISE) ARISING IN ANY WAY OUT OF THE USE OF THIS SOFTWARE, EVEN IF ADVISED OF THE POSSIBILITY OF SUCH DAMAGE."
  n1 = call "AlliGator Event to String.vi"("AlliGator Q Event"="AlliGator Q Event in") -> ("String"=w9:string)  [unwired: 8 in]
  n2 = case shown="\"Parameter Map:Change Parameter Map Color Palette\"" "AlliGator Q Event in" {
    selector: "AlliGator Q Event in" -> [_ _ _ w83 _ _ _ _ _ _ _ _ _ _ _ _ _ _ _ _]
    tunnel: "Data" -> [_ w40 w45 w84 _ w140 _ w174 w190 w192 w208 _ w246 _ w307 w315 _ w368 w384 w401]
    tunnel: "AlliGator Q Elements in" -> [w22 w30 w61 w70 w136 w143 w158 w175 w191 w203 w211 w220 w256 w270 w309 w318 w353 w373 w393 w402]
    tunnel: [w22 w29 w60 w70 w136 w142 w158 w175 w191 w203 w210 w219 w256 w270 w309 w318 w353 w373 w393 w402] -> w11
    tunnel: "VI in" -> [_ _ w51 w65 _ _ w155 w167 w180 _ _ w217 w251 _ w272 w314 w348 w367 _ _]
    tunnel: "Script in" -> [w19 w42 w62 w64 w135 w144 w150 w162 w179 w202 w212 w215 w247 w266 w271 w311 w342 w362 w385 w395]
    tunnel: w9 -> [_ _ w43 w63 _ _ w156 w171 w182 _ _ w214 w254 _ w274 w316 w351 w371 _ _]
    tunnel: "error in (no error)" -> [w21 w31 _ w69 w130 w139 _ _ w185 w200 w205 _ _ w269 _ _ _ _ w383 _]
    tunnel: [w21 w27 w54 w66 w132 w141 w157 w172 w181 w201 w209 w216 w255 w269 w280 w317 w352 w372 w386 w396] -> w1
    tunnel: "AlliGator Ctrl Refnums" -> [_ w34 w53 w80 w129 _ w148 w169 w178 w199 _ w218 w252 _ w294 _ w349 w369 w391 _]
    tunnel: "data value reference" -> [w20 w41 w49 w77 w134 w145 w153 w165 w189 w197 w213 w222 w249 w268 w285 w312 w344 w364 w388 w399]
    tunnel: [w20 w41 w48 w77 w133 w145 w154 w166 w188 w196 w213 w221 w250 w268 w283 w313 w345 w365 w388 w398] -> w18
    tunnel: [_ _ _ w75 w131 _ w149 w161 w184 _ _ _ w244 _ w281 w310 w341 w359 w387 _] -> w6
    tunnel: [w19 w42 w62 w64 w135 w144 w150 w162 w179 w202 w212 w215 w247 w266 w271 w311 w342 w362 w385 w395] -> w8
    tunnel: [_ _ _ _ _ _ _ _ _ _ _ _ Text_Format_List."Result" ("Text Format") _ _ _ Text_Format_List."Result" ("Text Format") Text_Format_List."Result" ("Text Format") _ Text_Format_List."Message" ("Text Format")] -> w3
    frame "---- Parameter Map ----", Default {
    }
    frame "Parameter Map:Add Parameter Map Set" {
      # "Parameter Map:Add Parameter Map Set"
      n3 = Variant To Data(error in=w31, type=T18 {"New Parameter Set Name"="", "Parameter Map Names"=[]} ("New Parameter Map Set"), Variant=w40) -> (data=w37:T18, error out=w38:errorcluster)
      n4 = Unbundle By Name(w34) -> ("Parameter Map Ctrl Refnums.Parameter Map Set"=w33:refnum<vi>, "Parameter Map Ctrl Refnums.Map Parameter"=w32:refnum<vi>)
      n5 = Unbundle By Name(w37) -> ("New Parameter Set Name"=w36:string, "Parameter Map Names"=w35:string[])
      n6 = call "AlliGator Add New Parameter Map Set.vi"("Parameter Map Names"=w35, "error in (no error)"=w38, "Map Parameter Refnum"=w32, "New Parameter Map Set"=w36, "Parameter Map Set Refnum"=w33) -> ("error out"=w28:errorcluster, "Build Parameter Map Event Data"=w24:T33)  [unwired: 5 in]
      n7 = Bundle By Name(cluster=T6 {"AlliGator Q Event"=enum."Parameter Map:Build Parameter Map", "Data"=variant} ("Alligator Atomic Action"), "Data"=w24) -> (w25:T6)
      n8 = call-poly "AlliGator Add Action(s) to Stack.vi"("Elements Order in Action Stack (Default: 2 BEFORE 1)"=Alligator_Elements_Order_in_Action_Stack."Enqueue 2 BEFORE 1", "Error In"=w28, "Alligator Atomic Action"=w25, "Alligator Queue Element 1"=w30) -> ("Error Out"=w27:errorcluster, "Alligator Queue Element 1 (+ 2)"=w29:T6[])  [unwired: 6 in]
    }
    frame "Parameter Map:Build Parameter Map" {
      # "\"Build Parameter Map\""
      n9 = Unbundle By Name(w53) -> ("Parameter Map Ctrl Refnums"=w50:T16)
      n10 = Variant To Data(Variant=w45) -> (data=w46:T33, error out=w44:errorcluster)  [unwired: 2 in]
      n11 = call "Show Animated Busy Icon with Message.vi"("Already active? (F)"=w62, "Message"=w43, "Error In"=w44, "Target VI Refnum"=w51) -> ("Error Out"=w52:errorcluster)  [unwired: 7 in]
      n12 = call "AlliGator Build Parameter Map.vi"("error in (no error)"=w52, "Parameter Map Update Event Data"=w46, "Parameter Map Ctrl Refums"=w50, "AlliGator Internal Variables DVR"=w49) -> ("error out"=w59:errorcluster, "AlliGator Internal Variables DVR"=w48:refnum<data-value>)  [unwired: 3 in, 3 out]
      n13 = call "Hide Animated Busy Icon with Message.vi"("Already active? (F)"=w62, "Error In"=w59, "Target VI reference"=w51) -> ("Error Out"=w47:errorcluster)  [unwired: 8 in]
      n14 = Bundle By Name(cluster=T6 {"AlliGator Q Event"=enum."Parameter Map:Change Parameter Map Color Palette", "Data"=variant} ("Alligator Atomic Action"), "Data"="Refresh Image") -> (w55:T6)
      n15 = call-poly "AlliGator Add Action(s) to Stack.vi"("Elements Order in Action Stack (Default: 2 BEFORE 1)"=Alligator_Elements_Order_in_Action_Stack."Enqueue 2 BEFORE 1", "Error In"=w47, "Alligator Atomic Action"=w55, "Alligator Queue Element 1"=w61) -> ("Error Out"=w54:errorcluster, "Alligator Queue Element 1 (+ 2)"=w60:T6[])  [unwired: 6 in]
    }
    frame "Parameter Map:Change Parameter Map Color Palette" {
      w71 = AlliGator_Variables_List."Parameter Map:Palette List" ("Alligator Variable")
      # "\"Change Parameter Map Color Palette\""
      n16 = call "Alligator Variables Storage.vi"("Get(F)/Set"=FALSE, "AlliGator Variable"=w71, "Error In"=w69) -> ("Error Out"=w68:errorcluster, "Data out"=w74:variant)  [unwired: 6 in, 1 out]
      n17 = call-poly "Variant to Data.vi"("Variant"=w84) -> ("String"=w82:string)  [unwired: 8 in]
      n18 = call-poly "Variant to Data.vi"("Variant"=w74) -> ("String Array"=w72:string[])  [unwired: 8 in]
      n19 = call "Show Animated Busy Icon with Message.vi"("Already active? (F)"=w64, "Message"=w63, "Error In"=w68, "Target VI Refnum"=w65) -> ("Error Out"=w67:errorcluster)  [unwired: 7 in]
      n20 = Unbundle By Name(w80) -> ("Parameter Map Ctrl Refnums"=w79:T16)
      n21 = case shown="Default" w82 {
        selector: w82 -> [_ w112 _]
        tunnel: w83 -> [_ _ _]
        tunnel: [w90 w98 w125] -> w81
        tunnel: [w89 w95 w123] -> w78
        tunnel: ["Palette List Edited" ("Append to Message") w104 _] -> w75
        tunnel: w72 -> [w86 w102 _]
        tunnel: w71 -> [w85 w97 _]
        tunnel: w67 -> [_ w96 _]
        tunnel: w63 -> [_ w94 _]
        frame "Edit Palette List..." {
          n22 = call "Edit Image Palette List Dialog.vi"("Palette List (in)"=w86) -> ("Palette List (out)"=w93:string[])  [unwired: 10 in]
          n23 = call "Alligator Variables Storage.vi"("Get(F)/Set"=TRUE, "AlliGator Variable"=w85, "Data in"=w93) -> ("Error Out"=w91:errorcluster)  [unwired: 6 in, 2 out]
          n24 = call "AlliGator Check Selected Palette.vi"("Error In"=w91, "Image"=AlliGator_Image_Display_Type."Parameter Map") -> ("Error Out"=w90:errorcluster, "Image Display Palette Information"=w89:T21)  [unwired: 8 in]
        }
        frame Default {
          n25 = call "Get User Palette Choice.vi"("Error In"=w96, "Palette"=w112) -> ("Error Out"=w108:errorcluster, "Palette Colors"=w110:u32[], "Palette Type"=w111:T22, "Palette Name (# Colors)"=w100:string, "Interpolate?"=w106:bool, "Built-in Palette?"=w101:bool)  [unwired: 2 in, 2 out]
          n26 = Format Into String(format string=": %s", initial string=w94, w100) -> (resulting string=w104:string)  [unwired: 1 in, 1 out]
          n27 = Bundle(cluster=T21 {"Palette Name [# Colors,int?,inv?]"="", "Palette Type"=0, "Palette Colors"=[], "Interpolate?"=FALSE} ("Image Display Palette Information"), "Palette Name [# Colors,int?,inv?]"=w100, "Palette Type"=w111, "Palette Colors"=w110, "Interpolate?"=w106) -> (w95:T21)
          n28 = call "Alligator Variables Storage.vi"("Get(F)/Set"=TRUE, "AlliGator Variable"=AlliGator_Variables_List."Parameter Map:Palette Information" ("Alligator Variable"), "Error In"=w108, "Data in"=w95) -> ("Error Out"=w99:errorcluster)  [unwired: 5 in, 2 out]
          n29 = case shown="False" w101 {
            tunnel: w99 -> [w120 w121]
            tunnel: [w119 w121] -> w98
            tunnel: w100 -> [w118 _]
            tunnel: w102 -> [w117 _]
            tunnel: w97 -> [w113 _]
            frame False {
              n30 = Build Array (concatenate)(w117, w118) -> (w116:string[])
              n31 = call "Remove Duplicates From 1D Array.vim"("array"=w116) -> ("array with duplicates removed"=w115:string[])  [unwired: 10 in]
              n32 = call "Alligator Variables Storage.vi"("Get(F)/Set"=TRUE, "AlliGator Variable"=w113, "Error In"=w120, "Data in"=w115) -> ("Error Out"=w119:errorcluster)  [unwired: 5 in, 2 out]
            }
            frame True {
            }
          }
        }
        frame "Refresh Image" {
          n33 = call "Alligator Variables Storage.vi"("Get(F)/Set"=FALSE, "AlliGator Variable"=AlliGator_Variables_List."Parameter Map:Palette Information" ("Alligator Variable")) -> ("Error Out"=w126:errorcluster, "Data out"=w127:variant)  [unwired: 7 in, 1 out]
          n34 = Variant To Data(error in=w126, type=T21 {"Palette Name [# Colors,int?,inv?]"="", "Palette Type"=0, "Palette Colors"=[], "Interpolate?"=FALSE} ("Image Display Palette Information"), Variant=w127) -> (data=w123:T21, error out=w125:errorcluster)
        }
      }
      n35 = call "AlliGator Update Parameter Map Palette.vi"("error in (no error)"=w81, "Parameter Map Display Palette Information"=w78, "Parameter Map Ctrl Refums"=w79) -> ("error out"=w76:errorcluster)  [unwired: 8 in]
      n36 = call "Hide Animated Busy Icon with Message.vi"("Already active? (F)"=w64, "Error In"=w76, "Target VI reference"=w65) -> ("Error Out"=w66:errorcluster)  [unwired: 8 in]
    }
    frame "Parameter Map:Delete Parameter Map Set" {
      # "Parameter Map:Delete Parameter Map Set"
      n37 = call "AlliGator Delete Parameter Map Set.vi"("AlliGator Ctrl Refnums"=w129, "error in (no error)"=w130, "AlliGator IV DVR in"=w134) -> ("error out"=w132:errorcluster, "Message"=w131:string, "AlliGator IV DVR out"=w133:refnum<data-value>)  [unwired: 6 in]
    }
    frame "Parameter Map:Display Range Mouse Move" {
      # "\"Parameter Map:Display Range Mouse Move\""
      n38 = Variant To Data(error in=w139, Variant=w140) -> (data=w137:T34, error out=w138:errorcluster)  [unwired: 1 in]
      n39 = call "AlliGator Parameter Map Range Mouse Move Event.vi"("Error In"=w138, "Mouse Move Data"=w137, "AlliGator Actions in"=w143) -> ("Error Out"=w141:errorcluster, "AlliGator Actions out"=w142:T6[])  [unwired: 7 in]
    }
    frame "Parameter Map:Export All Parameter Maps Data as ASCII" {
      # "\"Export All Parameter Maps Data as ASCII\""
      n40 = Unbundle By Name(w148) -> ("Parameter Map Ctrl Refnums.Parameter Map Set"=w147:refnum<vi>)
      n41 = property class="Ring (strict)"(reference=w147) -> ("Value"=w146:u16)  [unwired: 1 in, 2 out]
      n42 = call "Show Animated Busy Icon with Message.vi"("Already active? (F)"=w150, "Message"=w156, "Target VI Refnum"=w155) -> ("Error Out"=w151:errorcluster)  [unwired: 8 in]
      n43 = call "AlliGator Save All Parameter Maps to ASCII.vi"("error in (no error)"=w151, "Parameter Map Set"=w146, "Data Value Reference in"=w153) -> ("error out"=w152:errorcluster, "Data Value Reference out"=w154:refnum<data-value>, "Message"=w149:string)  [unwired: 6 in]
      n44 = call "Hide Animated Busy Icon with Message.vi"("Already active? (F)"=w150, "Error In"=w152, "Target VI reference"=w155) -> ("Error Out"=w157:errorcluster)  [unwired: 8 in]
    }
    frame "Parameter Map:Export Parameter Map Data as ASCII" {
      # "\"Export Parameter Map Data as ASCII\""
      n45 = call-poly "Variant to Data.vi"("Variant"=w174) -> ("Value"=w173:bool)  [unwired: 8 in]
      n46 = Unbundle By Name(w169) -> ("Parameter Map Ctrl Refnums.Parameter Map Set"=w160:refnum<vi>, "Parameter Map Ctrl Refnums.Map Parameter"=w170:refnum<vi>)
      n47 = property class="Ring (strict)"(reference=w160) -> ("Value"=w159:u16)  [unwired: 1 in, 2 out]
      n48 = property class="Ring (strict)"(reference=w170) -> ("Value"=w168:u16)  [unwired: 1 in, 2 out]
      n49 = call "Show Animated Busy Icon with Message.vi"("Already active? (F)"=w162, "Message"=w171, "Target VI Refnum"=w167) -> ("Error Out"=w164:errorcluster)  [unwired: 8 in]
      n50 = call "AlliGator Save Parameter Map to ASCII.vi"("Dialog?"=w173, "error in (no error)"=w164, "Parameter"=w168, "Map Set"=w159, "Data Value Reference in"=w165) -> ("error out"=w163:errorcluster, "Data Value Reference out"=w166:refnum<data-value>, "Message"=w161:string)  [unwired: 4 in]
      n51 = call "Hide Animated Busy Icon with Message.vi"("Already active? (F)"=w162, "Error In"=w163, "Target VI reference"=w167) -> ("Error Out"=w172:errorcluster)  [unwired: 8 in]
    }
    frame "Parameter Map:Export ROI Parameters Data as ASCII" {
      # "Export ROI Parameters Data as ASCII"
      n52 = call-poly "Variant to Data.vi"("Variant"=w190) -> ("Value"=w187:bool)  [unwired: 8 in]
      n53 = Unbundle By Name(w178) -> ("Parameter Map Ctrl Refnums.Parameter Map Set"=w177:refnum<vi>)
      n54 = property class="Ring (strict)"(reference=w177) -> ("Value"=w176:u16)  [unwired: 1 in, 2 out]
      n55 = call "Show Animated Busy Icon with Message.vi"("Already active? (F)"=w179, "Message"=w182, "Error In"=w185, "Target VI Refnum"=w180) -> ("Error Out"=w183:errorcluster)  [unwired: 7 in]
      n56 = call "AlliGator Export ROI(s) Parameter Set as ASCII File.vi"("error in (no error)"=w183, "Parameter Map Set"=w176, "All ROIs"=w187, "AlliGator IV DVR in"=w189) -> ("error out"=w186:errorcluster, "Message"=w184:string, "AlliGator IV DVR out"=w188:refnum<data-value>)  [unwired: 5 in]
      n57 = call "Hide Animated Busy Icon with Message.vi"("Already active? (F)"=w179, "Error In"=w186, "Target VI reference"=w180) -> ("Error Out"=w181:errorcluster)  [unwired: 8 in]
    }
    frame "Parameter Map:Mouse Move" {
      # "\"Parameter Map:Mouse Move\""
      n58 = Unbundle By Name(w199) -> ("Parameter Map Ctrl Refnums"=w198:T16, "Registered Events Ctrl Refnums.Parameter Map Display"=w193:refnum<vi>)
      n59 = call "AlliGator Display Current Parameter Map (X,Y, I).vi"("Parameter Map Ctrl Refums"=w198, "error in (no error)"=w200, "AlliGator Internal Variables DVR"=w197) -> ("error out"=w201:errorcluster, "AlliGator Internal Variables DVR"=w196:refnum<data-value>)  [unwired: 7 in]
      n60 = call-poly "Variant to Data.vi"("Variant"=w192) -> ("Value"=w195:bool)  [unwired: 8 in]
      n61 = call "AlliGator Generic Image Display Mouse Move Flag.vi"("Image Control Refnum"=w193, "Flag (in)"=w195, "Read/Write"=Read-Write."Write") -> ()  [unwired: 6 in, 1 out]
    }
    frame "Parameter Map:Mouse Up" {
      # "\"Parameter Map:Mouse Up\""
      n62 = Variant To Data(error in=w205, type=T24 {"Current ROI Tool"=8, "ROI Descriptor"={"Global Rectangle"=[], "Contours"=[]}, "Shift"=FALSE, "Alt"=FALSE, "Image Display Refnum"=refnum} ("Phasor Plot Mouse Up Event Data"), Variant=w208) -> (data=w207:T24, error out=w206:errorcluster)
      n63 = call "AlliGator Parameters Map Mouse Up Event.vi"("error in (no error)"=w206, "Image Mouse Up Event Data"=w207, "AlliGator Actions in"=w211) -> ("error out"=w209:errorcluster, "AlliGator Actions out"=w210:T6[])  [unwired: 7 in]
    }
    frame "Parameter Map:Overlay Parameter Map in Source Image" {
      # "\"Overlay Parameter Map in Source Image\""
      n64 = Unbundle By Name(w218) -> ("Dataset Control Refnums.Save Image"=w226:refnum<vi>)
      n65 = Unbundle By Name(w218) -> ("Parameter Map Ctrl Refnums.Parameter Map Color Scale"=w228:refnum<vi>, "Dataset Control Refnums.Image Color Scale"=w229:refnum<vi>, "Registered Events Ctrl Refnums.Source Image Display"=w227:refnum<vi>)
      n66 = property class="Bool (strict)"(reference=w226) -> ("Value"=w225:bool)  [unwired: 1 in, 2 out]
      n67 = case shown="True" w225 {
        tunnel: w220 -> [w230 w234]
        tunnel: [w230 w231] -> w219
        frame False {
        }
        frame True {
          n68 = call-poly "AlliGator Add Action(s) to Stack.vi"("Elements Order in Action Stack (Default: 2 BEFORE 1)"=Alligator_Elements_Order_in_Action_Stack."Enqueue 2 BEFORE 1", "Alligator Atomic Action"=T6 {"AlliGator Q Event"=enum."Image:Save Displayed Image with Overlay", "Data"=variant}, "Alligator Queue Element 1"=w234) -> ("Alligator Queue Element 1 (+ 2)"=w231:T6[])  [unwired: 7 in, 1 out]
        }
      }
      n69 = call "Show Animated Busy Icon with Message.vi"("Already active? (F)"=w215, "Message"=w214, "Target VI Refnum"=w217) -> ("Error Out"=w224:errorcluster)  [unwired: 8 in]
      n70 = call "AlliGator Color Parameter Map in Original Image.vi"("Color Scale Refnum"=w228, "Image Color Scale Refnum"=w229, "Error In"=w224, "Destination Image Control Refnum"=w227, "AlliGator IV DVR in"=w222) -> ("Error Out"=w223:errorcluster, "AlliGator IV DVR out"=w221:refnum<data-value>)  [unwired: 4 in, 1 out]
      n71 = call "Hide Animated Busy Icon with Message.vi"("Already active? (F)"=w215, "Error In"=w223, "Target VI reference"=w217) -> ("Error Out"=w216:errorcluster)  [unwired: 8 in]
    }
    frame "Parameter Map:Parameter 2 vs Parameter 1 Scatterplot" {
      # "Parameter 2 vs Parameter 1 Scatterplot"
      n72 = call "Show Animated Busy Icon with Message.vi"("Already active? (F)"=w247, "Message"=w254, "Target VI Refnum"=w251) -> ("Error Out"=w245:errorcluster)  [unwired: 8 in]
      n73 = Variant To Data(error in=w245, type=T31 {"Parameter Map Set"=0, "Map Parameter 1"=0, "Map Parameter 2"=0}, Variant=w246) -> (data=w241:T31, error out=w242:errorcluster)
      n74 = Unbundle By Name(w252) -> ("Registered Events Ctrl Refnums.Lifetime Graph"=w253:refnum<vi>, "Parameter Map Ctrl Refnums.Parameter Map Set"=w237:refnum<vi>)
      n75 = case shown="Error .." w242 {
        selector: w242 -> [w257 _]
        tunnel: w241 -> [w261 _]
        tunnel: [w260 w265] -> w240
        tunnel: [w259 w265] -> w239
        tunnel: [w258 w263] -> w238
        tunnel: w237 -> [_ w264]
        tunnel: [w257 w262] -> w235
        frame No Error {
          n76 = Unbundle By Name(w261) -> ("Map Parameter 1"=w260:u16, "Map Parameter 2"=w259:u16, "Parameter Map Set"=w258:u16)
        }
        frame Error {
          w265 = u16 0 ("Map Parameter 1")
          n77 = property class="Ring (strict)"(reference=w264) -> (error out=w262:errorcluster, "Value"=w263:u16)  [unwired: 1 in, 1 out]
        }
      }
      n78 = call "AlliGator Plot Parameter 2 vs Parameter 1.vi"("Parameter Map Set"=w238, "Lifetime Graph refnum"=w253, "error in (no error)"=w235, "Map Parameter 2"=w239, "Map Parameter 1"=w240, "Data Value Reference in"=w249) -> ("error out"=w248:errorcluster, "Data Value Reference out"=w250:refnum<data-value>, "Message"=w244:string)  [unwired: 3 in]
      n79 = call "Hide Animated Busy Icon with Message.vi"("Already active? (F)"=w247, "Error In"=w248, "Target VI reference"=w251) -> ("Error Out"=w255:errorcluster)  [unwired: 8 in]
    }
    frame "Parameter Map:Python Function Parameter Map Event" {
      # "\"Parameters:Python Function Parameter Map Event\""
      n80 = One Button Dialog(message="Not yet supported....") -> ()  [unwired: 1 in, 1 out]
      n81 = call "Play Error Sound.vi"() -> ()  [unwired: 27 in, 1 out]
    }
    frame "Parameter Map:Save Parameter Map Image" {
      # "\"Save Parameter Map Image\""
      n82 = Unbundle By Name(w294) -> ("Parameter Map Ctrl Refnums.Parameter Map Display"=w308:refnum<vi>, "Parameter Map Ctrl Refnums.Map Parameter"=w293:refnum<vi>)
      n83 = call-poly "Variant to Data.vi"("Variant"=w307) -> ("Value"=w301:bool)  [unwired: 8 in]
      n84 = call "AlliGator IV Dataset Path.vi"("Get (F)/ Set (T)"=FALSE, "AlliGator IV DVR in"=w285) -> ("error out"=w282:errorcluster, "[Time-Series Path]"=w287:path[], "Single Data Point Path"=w288:path, "AlliGator IV DVR out"=w283:refnum<data-value>, "Current Dataset"=w286:i32)  [unwired: 5 in]
      n85 = call "Show Animated Busy Icon with Message.vi"("Already active? (F)"=w271, "Message"=w274, "Error In"=w282, "Target VI Refnum"=w272) -> ("Error Out"=w275:errorcluster)  [unwired: 7 in]
      n86 = property class="Ring (strict)"(reference=w293) -> ("Strings []"=w278:string[], "Value"=w277:u16)  [unwired: 1 in, 2 out]
      n87 = call "AlliGator Get Image File Format.vi"("Error In"=w275) -> ("error out"=w298:errorcluster, "Transparent Mask Color"=w279:u32, "File Extension (.xxx)"=w295:string, "Image File Format"=w303:T35)  [unwired: 7 in]
      n88 = call "AlliGator Get Destination Folder.vi"("Current Data Set (-1: single)"=w286, "Time-Series Paths"=w287, "Single Data Point Path"=w288) -> ("Data Point Name"=w300:string, "Destination Folder path"=w306:path)  [unwired: 5 in, 2 out]
      n89 = Index Array(array=w278, index=w277) -> (element=w276:string)
      n90 = Format Into String(format string=" %s Map%s", initial string=w300, error in=w298, w276, w295) -> (resulting string=w297:string, error out=w296:errorcluster)
      n91 = Build Path(base path=w306, name or relative path=w297) -> (appended path=w305:path)
      n92 = call "Image File Dialog (Optional).vi"("Dialog?"=w301, "Error In"=w296, "Image File Format in"=w303, "Default file path in"=w305) -> ("Error Out"=w289:errorcluster, "Image File Format out"=w302:T35, "file path out"=w304:path)  [unwired: 5 in]
      n93 = call "Image Display Save Image.vi"("Mask Color (Transparent)"=w279, "error in (no error)"=w289, "Saved Image File Format"=w302, "File Path in"=w304, "Display Image Control Refnum"=w308) -> ("Error Out"=w290:errorcluster, "File Path out"=w291:path)  [unwired: 5 in]
      n94 = call "Hide Animated Busy Icon with Message.vi"("Already active? (F)"=w271, "Error In"=w290, "Target VI reference"=w272) -> ("Error Out"=w273:errorcluster)  [unwired: 8 in]
      n95 = Format Into String(format string="Parameter Map Image saved to %s", error in=w273, w291) -> (resulting string=w281:string, error out=w280:errorcluster)  [unwired: 1 in]
    }
    frame "Parameter Map:Save-Load IRFs & Parameter Maps (TODO)" {
      # "Save-Load IRFs & Parameter Maps (TODO)"
      n96 = disable-structure shown="Enabled" {
        disable-tunnel: [w332 _] -> w317
        disable-tunnel: w316 -> [w331 _]
        disable-tunnel: w315 -> [w330 _]
        disable-tunnel: w314 -> [w325 _]
        disable-tunnel: [w324 w334] -> w313
        disable-tunnel: w312 -> [w323 w334]
        disable-tunnel: w311 -> [w320 _]
        disable-tunnel: [w319 _] -> w310
        frame Disabled {
          n97 = Variant To Data(type=T32 {"Load/Save"=FALSE, "File Path"=path ""} ("Calibration File Information"), Variant=w330) -> (data=w328:T32)  [unwired: 1 in, 1 out]
          n98 = Unbundle By Name(w328) -> ("File Path"=w327:path, "Load/Save"=w326:bool)
          n99 = call "Show Animated Busy Icon with Message.vi"("Already active? (F)"=w320, "Message"=w331, "Target VI Refnum"=w325) -> ("Error Out"=w322:errorcluster)  [unwired: 8 in]
          n100 = call "AlliGator Save-Load IRFs & Fit Data (Map).vi"("error in (no error)"=w322, "Write(T)/Load (F)"=w326, "File Path"=w327, "Data Value Reference in"=w323) -> ("error out"=w321:errorcluster, "Data Value Reference out"=w324:refnum<data-value>, "Message"=w319:string)  [unwired: 5 in]
          n101 = call "Hide Animated Busy Icon with Message.vi"("Already active? (F)"=w320, "Error In"=w321, "Target VI reference"=w325) -> ("Error Out"=w332:errorcluster)  [unwired: 8 in]
        }
        frame Enabled {
          n102 = One Button Dialog(message="Not yet implemented!") -> ()  [unwired: 1 in, 1 out]
        }
      }
    }
    frame "Parameter Map:Selected Parameter Scatterplot" {
      # "Selected Parameter Scatterplot"
      n103 = Unbundle By Name(w349) -> ("Registered Events Ctrl Refnums.Lifetime Graph"=w350:refnum<vi>, "Parameter Map Ctrl Refnums.Parameter Map Set"=w347:refnum<vi>, "Parameter Map Ctrl Refnums.Map Parameter"=w339:refnum<vi>)
      n104 = property class="Ring (strict)"(reference=w339) -> ("Strings []"=w338:string[], "Value"=w337:u16)  [unwired: 1 in, 2 out]
      n105 = property class="Ring (strict)"(reference=w347) -> ("Value"=w340:u16)  [unwired: 1 in, 2 out]
      n106 = Index Array(array=w338, index=w337) -> (element=w336:string)
      n107 = call "Show Animated Busy Icon with Message.vi"("Already active? (F)"=w342, "Message"=w351, "Target VI Refnum"=w348) -> ("Error Out"=w346:errorcluster)  [unwired: 8 in]
      n108 = call "AlliGator Plot Parameter Scatterplot.vi"("Lifetime Graph refnum"=w350, "error in (no error)"=w346, "Map Parameter"=w336, "Parameter Map Set"=w340, "Data Value Reference in"=w344) -> ("error out"=w343:errorcluster, "Data Value Reference out"=w345:refnum<data-value>, "Message"=w341:string)  [unwired: 4 in]
      n109 = call "Hide Animated Busy Icon with Message.vi"("Already active? (F)"=w342, "Error In"=w343, "Target VI reference"=w348) -> ("Error Out"=w352:errorcluster)  [unwired: 8 in]
    }
    frame "Parameter Map:Selected Parameter vs Intensity Scatterplot" {
      # "Selected Parameter vs Intensity Scatterplot"
      n110 = call-poly "Variant to Data.vi"("Variant"=w368) -> ("Value"=w355:i32)  [unwired: 8 in]
      n111 = Unbundle By Name(w369) -> ("Registered Events Ctrl Refnums.Lifetime Graph"=w370:refnum<vi>, "Parameter Map Ctrl Refnums.Parameter Map Set"=w366:refnum<vi>, "Parameter Map Ctrl Refnums.Map Parameter"=w358:refnum<vi>)
      n112 = property class="Ring (strict)"(reference=w366) -> ("Value"=w357:u16)  [unwired: 1 in, 2 out]
      n113 = property class="Ring (strict)"(reference=w358) -> ("Value"=w356:u16)  [unwired: 1 in, 2 out]
      n114 = call "Show Animated Busy Icon with Message.vi"("Already active? (F)"=w362, "Message"=w371, "Target VI Refnum"=w367) -> ("Error Out"=w361:errorcluster)  [unwired: 8 in]
      n115 = disable-structure shown="Enabled" {
        disable-tunnel: w361 -> [w378 w379]
        disable-tunnel: [w377 w379] -> w360
        frame Disabled {
          n116 = call "Two Button Dialog with Error.vi"("Error In"=w378, "F button name (\"Cancel\")"="No" ("F button name (\"Cancel\")"), "T button name (\"OK\")"="Yes" ("T button name (\"OK\")"), "message"="Use baseline-subtracted intensity?") -> ("Error Out"=w377:errorcluster)  [unwired: 6 in, 1 out]
        }
        frame Enabled {
        }
      }
      n117 = call "AlliGator Plot Parameter vs Intensity Scatterplot v2.vi"("ROI idx (2147483647: all ROIs)"=w355, "Lifetime Graph refnum"=w370, "error in (no error)"=w360, "Parameter"=w356, "Map Parameter Set"=w357, "Data Value Reference in"=w364) -> ("error out"=w363:errorcluster, "Data Value Reference out"=w365:refnum<data-value>, "Message"=w359:string)  [unwired: 3 in]
      n118 = call "Hide Animated Busy Icon with Message.vi"("Already active? (F)"=w362, "Error In"=w363, "Target VI reference"=w367) -> ("Error Out"=w372:errorcluster)  [unwired: 8 in]
    }
    frame "Parameter Map:Set Parameter Map Selection" {
      # "used in script"
      # "\"Parameter Map:Set Parameter Map Selection\""
      n119 = Unbundle By Name(w391) -> ("Parameter Map Ctrl Refnums.Map Parameter"=w390:refnum<vi>)
      n120 = call-poly "Variant to Data.vi"("Variant"=w384) -> ("U16 Value"=w381:u16)  [unwired: 8 in]
      n121 = property class="Ring (strict)"(reference=w390, error in=w383, "Value"=w381) -> (error out=w389:errorcluster, "Strings []"=w382:string[])  [unwired: 1 out]
      n122 = Index Array(array=w382, index=w381) -> (element=w380:string)
      n123 = Format Into String(format string="Parameter Map Selection set to %s", error in=w389, w380) -> (resulting string=w387:string, error out=w386:errorcluster)  [unwired: 1 in]
    }
    frame "Parameter Map:Update Local Decay Plots" {
      # "\"Update Local Decay Plots\""
      n124 = Variant To Data(Variant=w401) -> (data=w400:T36, error out=w397:errorcluster)  [unwired: 2 in]
      n125 = call "AlliGator Send Local Decay Plots (Parameter Map).vi"("error in (no error)"=w397, "ROI Descriptor"=w400, "AlliGator IV DVR in"=w399) -> ("error out"=w396:errorcluster, "AlliGator IV DVR out"=w398:refnum<data-value>)  [unwired: 7 in]
    }
  }
  "Data Value Reference out" <- w18
  "error out" <- w1
  "AlliGator Q Elements out" <- w11
  "Script out" <- w8
  n126 = call "Get Current Message Text Format.vi"("Text Format"=w3) -> ("Error Out"=w2:errorcluster, "Message Formatting"=w5:T2)  [unwired: 8 in]
  n127 = call "AlliGator Package Notebook Messages.vi"("Error In"=w2, "Message Formatting"=w5, "Message"=w6, "AlliGator Q Event in"="AlliGator Q Event in") -> ("[Notebook Message]"=→"[Notebook Message]":T1[])  [unwired: 6 in, 1 out]
